vi "compare.add.data.to.buffer.results.vi"(9 "Test Case":T1={"data.valid"=FALSE, "buffer"=[0, 0, 0, 0, 0, 0, 0, 0, 0], "buffer.length"=0, "exp.buffer.value.1"=0, "index 1"=0, "exp.buffer.value.2"=0, "index 2"=0, "exp.buffer.length"=0, "Key (U64)"=0} {"index 2" format="%.0x"; "index 1" format="%.0x"; "buffer" format="%.0x"}, 10 "buffer.out":u64[](array[numeric])=[0, 0, 0, 0, 0, 0, 0, 0, 0], 11 "buffer.length.out":u8) -> (3 "All Passed":bool)   [LabVIEW 2020]
uses:
  Market.Data.Filter/fpga/tests/crc.test.case.ctl
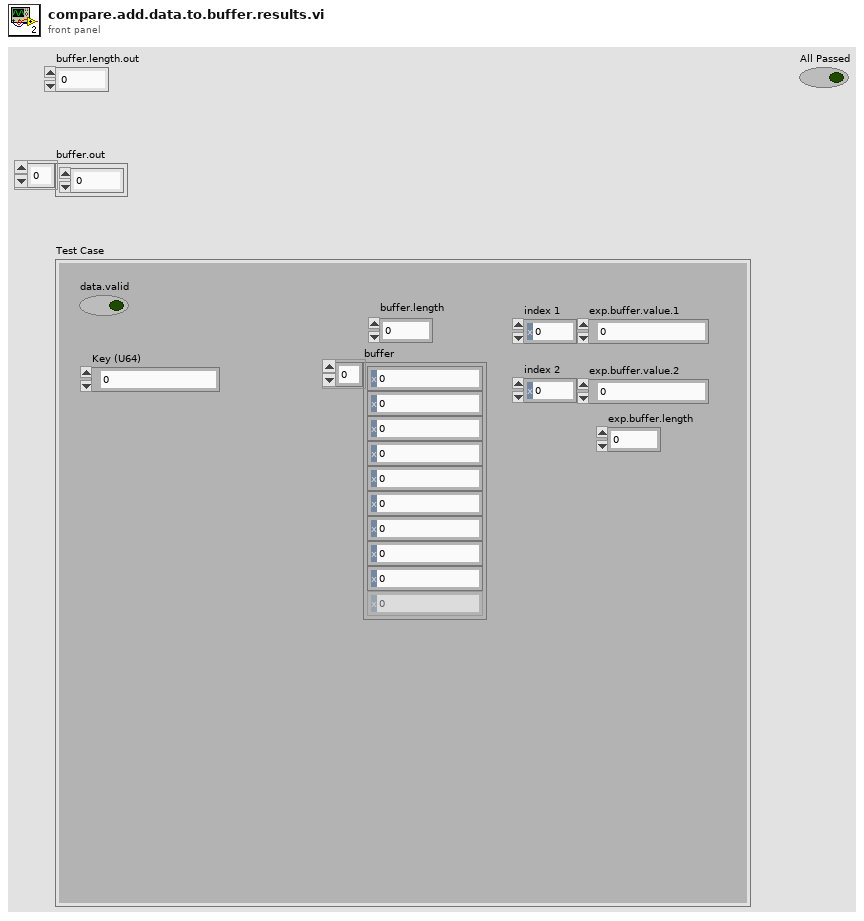
[diagram p1: front panel]
types:
  T1 = typedef "crc.test.case.ctl" = cluster{"data.valid":bool, "buffer":u64[], "buffer.length":u8, "exp.buffer.value.1":u64, "index 1":i16, "exp.buffer.value.2":u64, "index 2":i16, "exp.buffer.length":u8, "Key (U64)":u64}
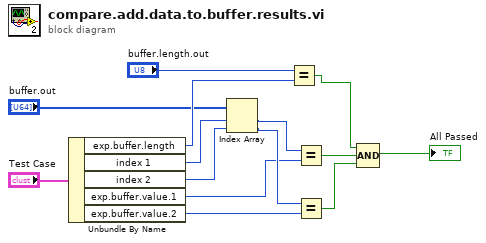
[diagram p0: block diagram]
diagram:
  n1 = Unbundle By Name("Test Case") -> ("exp.buffer.length"=w13:u8, "index 1"=w2:i16, "index 2"=w6:i16, "exp.buffer.value.1"=w7:u64, "exp.buffer.value.2"=w10:u64)
  n2 = Index Array(array="buffer.out", index #1=w2, index #2=w6) -> (element #1=w4:u64, element #2=w9:u64)
  n3 = Equal?(x="buffer.length.out", y=w13) -> (x = y?=w14:bool)
  n4 = Equal?(x=w4, y=w7) -> (x = y?=w5:bool)
  n5 = Equal?(x=w9, y=w10) -> (x = y?=w11:bool)
  n6 = Compound Arithmetic op=AND(w14, w5, w11) -> (→"All Passed":bool)
